vi "read_environment (SubVI).vi"(8 "data tasks":T1, 10 "Read pressures?":bool, 11 "Read temps?":bool) -> (0 "data tasks out":T1, 3 "environ cluster":cluster{dbl[], dbl[]})   [LabVIEW 2014]
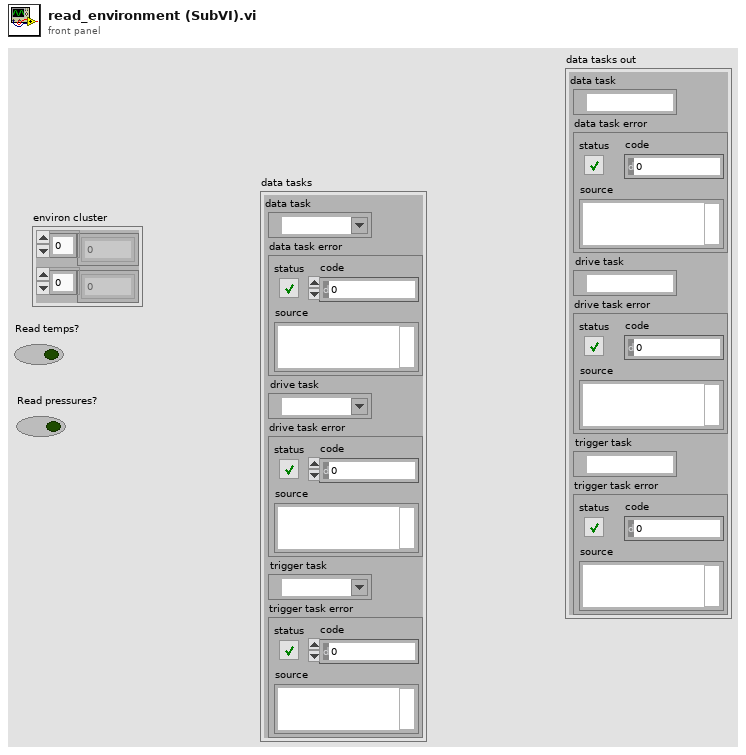
[diagram p1: front panel]
types:
  T1 = cluster{"data task":refnum<k21>, "data task error":errorcluster, "drive task":refnum<k21>, "drive task error":errorcluster, "trigger task":refnum<k21>, "trigger task error":errorcluster}
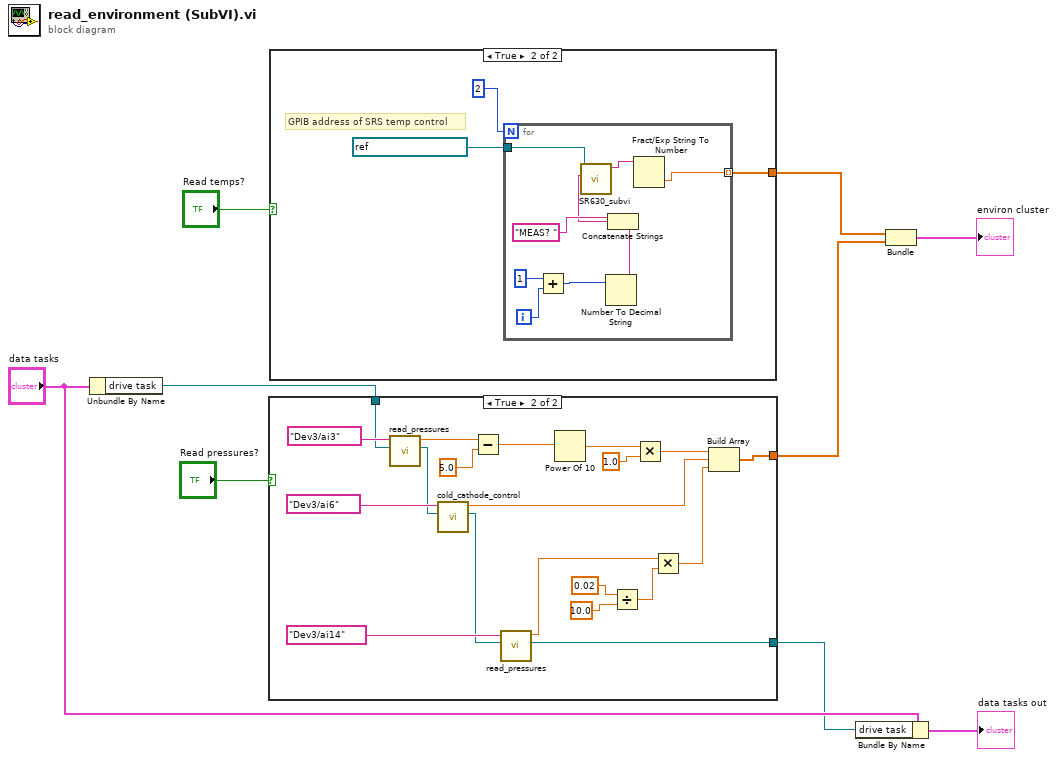
[diagram p0: block diagram]
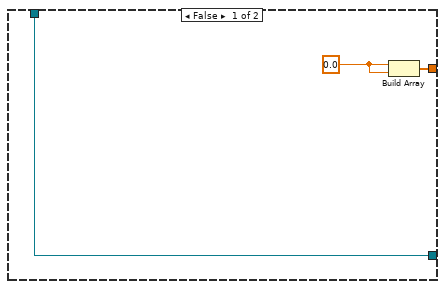
[diagram p2: hidden frame]
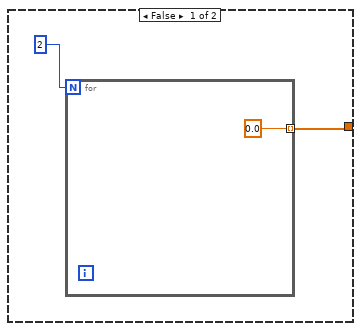
[diagram p3: hidden frame]
diagram:
  n1 = Unbundle By Name("data tasks") -> ("drive task"=w4:refnum<k21>)
  n2 = case shown="True" "Read pressures?" {
    tunnel: [w12 w23] -> w7
    tunnel: w4 -> [w10 w22]
    tunnel: [w10 w18] -> w2
    frame False {
      w11 = 0.0 ("element")
      n3 = Build Array(w11, w11) -> (w12:dbl[])
    }
    frame True {
      n4 = call "read_pressures.vi"("press task in"=w22, "Channel 1"=tag "Dev3/ai3") -> ("press task out"=w21:refnum<k21>, "Ch. 1 value"=w31:dbl)  [unwired: 8 in]
      n5 = call "cold_cathode_control.vi"("press task in"=w21, "Cold Cathode Gauge Channel"=tag "Dev3/ai6") -> ("press task out"=w19:refnum<k21>, "Cold Cathode Gauge Pressure"=w24:dbl)  [unwired: 8 in]
      n6 = Subtract(x=w31, y=5.0) -> (x-y=w30:dbl)
      n7 = call "read_pressures.vi"("press task in"=w19, "Channel 1"=tag "Dev3/ai14" ("Cold Cathode Gauge Channel")) -> ("press task out"=w18:refnum<k21>, "Ch. 1 value"=w14:dbl)  [unwired: 8 in]
      n8 = Power Of 10(x=w30) -> (10^x=w29:dbl)
      n9 = Divide(x=0.02, y=10.0) -> (x/y=w15:dbl)
      n10 = Multiply(x=w29, y=1.0) -> (x*y=w25:dbl)
      n11 = Multiply(x=w14, y=w15) -> (x*y=w13:dbl)
      n12 = Build Array(w25, w24, w13) -> (w23:dbl[])
    }
  }
  n13 = case shown="True" "Read temps?" {
    tunnel: [w33 w36] -> w6
    frame False {
      n14 = for {
        N: 2 ("dimension size") -> [_]
        tunnel: [0.0] -> w33 mode=indexing
      }
    }
    frame True {
      # "GPIB address of SRS temp control"
      n15 = for {
        N: 2 ("dimension size") -> [_]
        tunnel: refnum<visa-resource-name> "GPIB0::19::INSTR" ("VISA Refnum in") -> [w47]
        tunnel: [w45] -> w36 mode=indexing
        i -> [w44]
        n16 = Add(x=1, y=w44) -> (x+y=w42:i32)
        n17 = Number To Decimal String(number=w42) -> (decimal integer string=w41:string)  [unwired: 1 in]
        n18 = Concatenate Strings("MEAS? " ("Write Buffer"), w41) -> (w39:string)
        n19 = call "SR630_subvi.vi"("Write Buffer"=w39, "VISA Refnum in"=w47) -> ("read buffer"=w46:string)  [unwired: 9 in]
        n20 = Fract/Exp String To Number(string=w46) -> (number=w45:dbl)  [unwired: 3 in, 1 out]
      }
    }
  }
  n21 = Bundle By Name(cluster="data tasks", "drive task"=w2) -> (→"data tasks out":T1)
  n22 = Bundle(w6, w7) -> (→"environ cluster":cluster{dbl[], dbl[]})  [unwired: 1 in]
